vi "State Process.vi"(8 "error in (no error)":errorcluster, 11 "View Model":T1) -> (0 "error out":errorcluster, 3 "View Model":T1)   [LabVIEW 2017]
doc: "Provide processing current ATM controller state"
uses:
  View Model/Controls/View Model.ctl
  View Model/Controls/Shared Model.ctl
  Error Handler/Controls/Error Model.ctl
  Error Handler/Controls/Error Data.ctl
  Error Handler/Controls/Error Type.ctl
  Error Handler/Controls/Error Source.ctl
  Configuration/Controls/Config Model.ctl
  Configuration/Controls/Config CMD.ctl
  Configuration/Controls/Config Command.ctl
  Controls/Controller Model.ctl
  Controls/Controller Overhead.ctl
  Controls/Controller Transaction.ctl
  Controls/Controller State.ctl
  Configuration/Controls/Config Data Record.ctl
  Controls/Controller Message Selector.ctl
  Controls/Controller Message Type.ctl
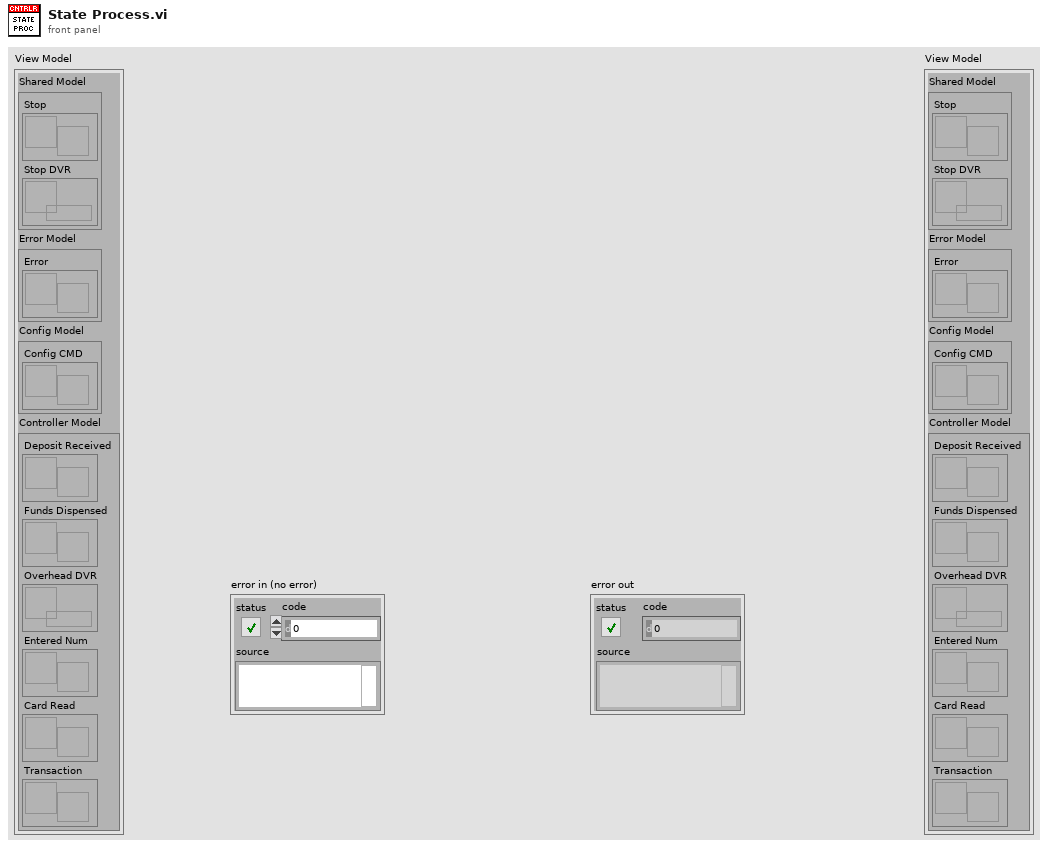
[diagram p1: front panel]
types:
  T1 = typedef "View Model.ctl" = cluster{"Shared Model":T2, "Error Model":T3, "Config Model":T4, "Controller Model":T5}
  T2 = typedef "Shared Model.ctl" = cluster{"Stop":refnum<user-event>, "Stop DVR":refnum<data-value>}
  T3 = typedef "Error Model.ctl" = cluster{"Error":refnum<user-event>}
  T4 = typedef "Config Model.ctl" = cluster{"Config CMD":refnum<user-event>}
  T5 = typedef "Controller Model.ctl" = cluster{"Deposit Received":refnum<user-event>, "Funds Dispensed":refnum<user-event>, "Overhead DVR":refnum<data-value>, "Entered Num":refnum<user-event>, "Card Read":refnum<user-event>, "Transaction":refnum<user-event>}
  T6 = typedef "Controller State.ctl" = enum16{"Idle", "Initial", "Login", "Balance Inquiry", "Deposit", "Withdrawal", "Fast Cash", "Terminate"}
  T7 = typedef "Controller Message Selector.ctl" = cluster{"Message Type":T8, "Dynamic Data":variant}
  T8 = typedef "Controller Message Type.ctl" = enum16{"Welcome", "Login", "Idle", "Invalid Login", "Terminate Session", "Deposit", "Withdrawal", "Fast Cash", "Withdrawal Complete", "Withdrawal Failed", "Balance"}
  T9 = typedef "Config Command.ctl" = enum16{"Read", "Search", "Update"}
  T10 = typedef "Config Data Record.ctl" = cluster{"Account Number":u32, "First Name":string, "Last Name":string, "Balance":dbl}
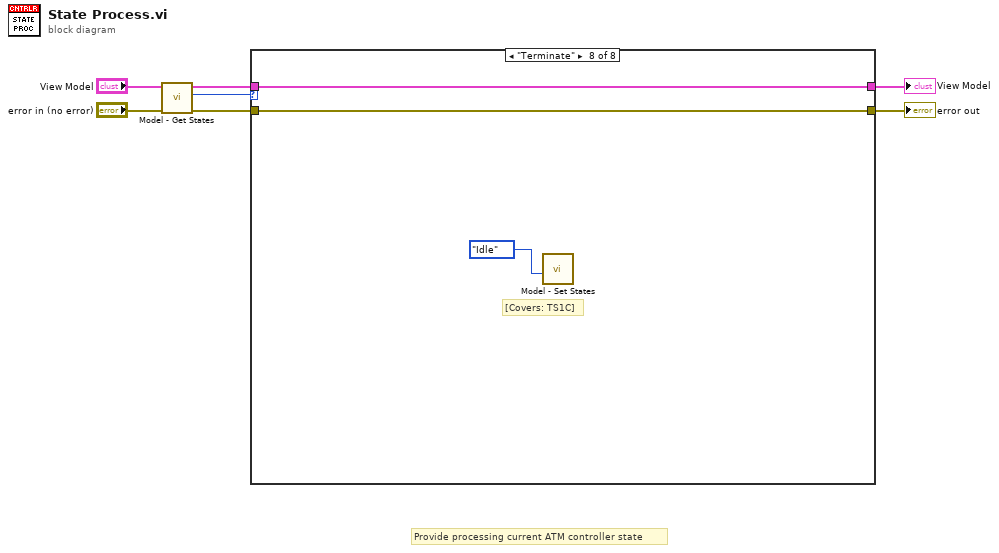
[diagram p0: block diagram]
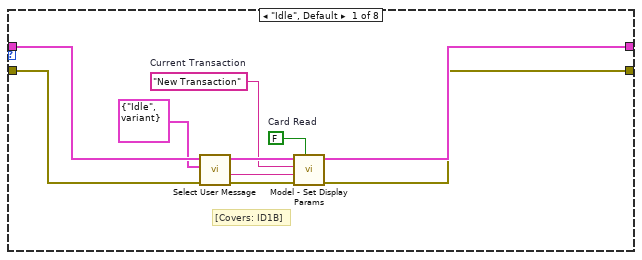
[diagram p2: hidden frame]
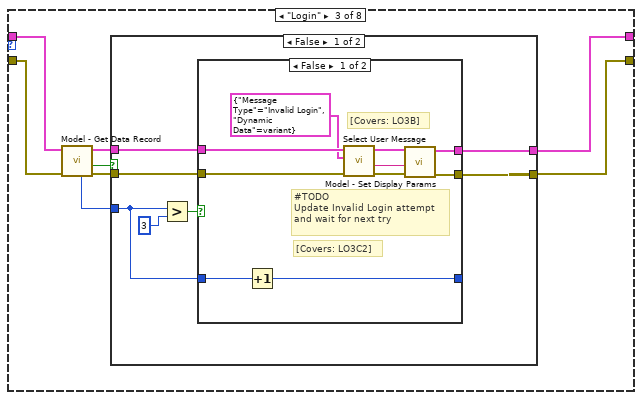
[diagram p4: hidden frame]
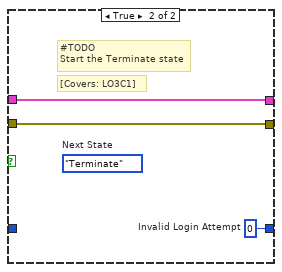
[diagram p5: hidden frame]
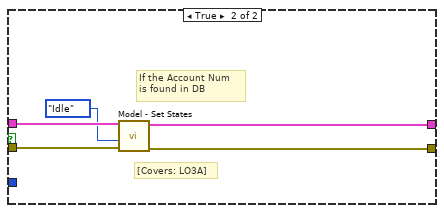
[diagram p6: hidden frame]
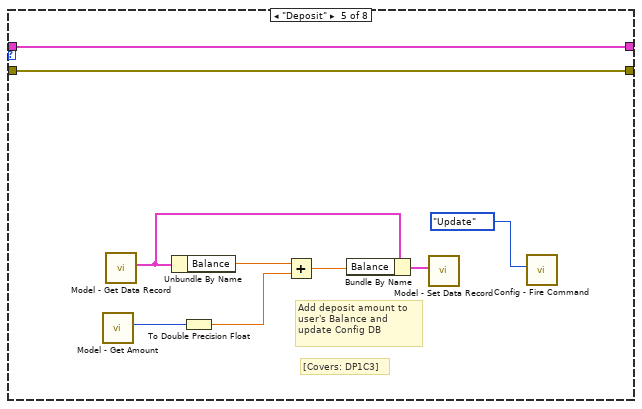
[diagram p8: hidden frame]
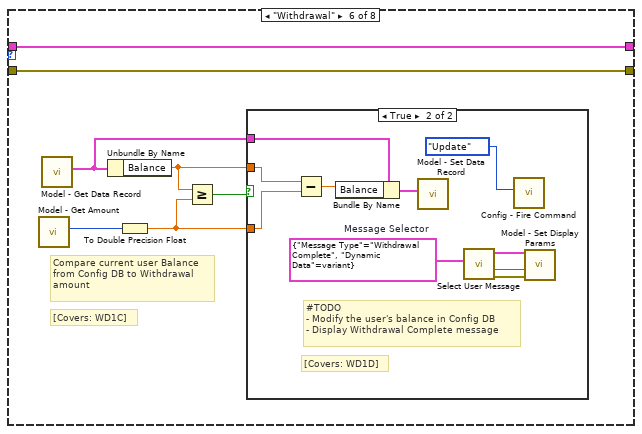
[diagram p9: hidden frame]
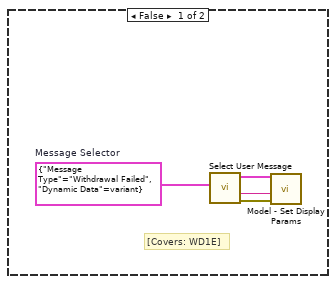
[diagram p10: hidden frame]
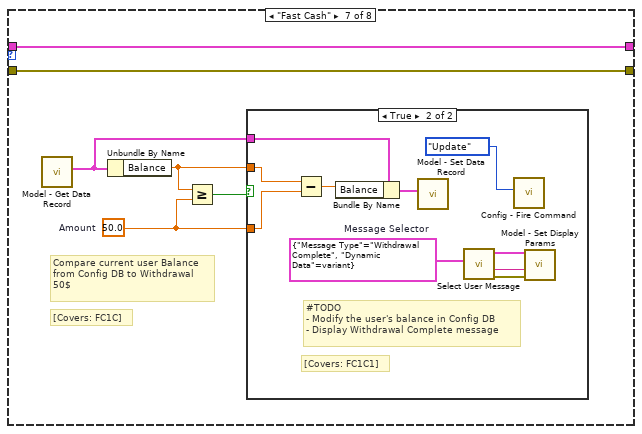
[diagram p11: hidden frame]
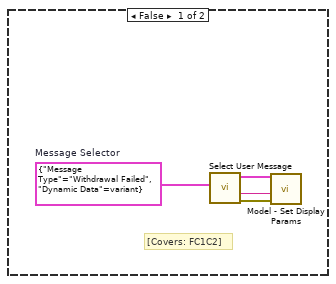
[diagram p12: hidden frame]
diagram:
  # "Provide processing current ATM controller state"
  n1 = call "Model - Get States.vi"("error in (no error)"="error in (no error)", "View Model"="View Model") -> ("error out"=w3:errorcluster, "Current State"=w5:T6, "View Model"=w4:T1)  [unwired: 6 in, 1 out]
  n2 = case shown="\"Terminate\"" w5 {
    tunnel: w4 -> [w16 w19 w26 w54 w63 w70 w90 w107]
    tunnel: w3 -> [w17 w18 w27 w53 w62 w69 w89 w106]
    tunnel: [w12 w19 w21 w54 w63 w70 w90 w107] -> w2
    tunnel: [w11 w18 w22 w53 w62 w69 w89 w106] -> w1
    frame "Idle", Default {
      w8 = FALSE  # Card Read
      w9 = "New Transaction"  # Current Transaction
      # "[Covers: ID1B]"
      n3 = call "Select User Message.vi"("error in (no error)"=w17, "Message Selector"=T7 {"Message Type"=enum."Idle", "Dynamic Data"=variant}, "View Model"=w16) -> ("error out"=w14:errorcluster, "Message"=w10:string, "View Model"=w13:T1)  [unwired: 6 in]
      n4 = call "Model - Set Display Params.vi"("Card Read"=w8, "error in (no error)"=w14, "Message"=w10, "Current Transaction"=w9, "View Model"=w13) -> ("error out"=w11:errorcluster, "View Model"=w12:T1)  [unwired: 5 in]
    }
    frame "Initial" {
    }
    frame "Login" {
      n5 = call "Model - Get Data Record.vi"("error in (no error)"=w27, "View Model"=w26) -> ("error out"=w23:errorcluster, "Account Found?"=w25:bool, "View Model"=w24:T1, "Invalid Login"=w20:u8)  [unwired: 5 in, 1 out]
      n6 = case shown="False" w25 {
        tunnel: w24 -> [w33 w51]
        tunnel: w23 -> [w34 w52]
        tunnel: [w32 w50] -> w22
        tunnel: [w31 w49] -> w21
        tunnel: w20 -> [w28 _]
        frame False {
          n7 = Greater?(x=w28, y=u8 3) -> (0:w30:bool)
          n8 = case shown="False" w30 {
            tunnel: w34 -> [w44 w47]
            tunnel: w33 -> [w43 w46]
            tunnel: [w40 w47] -> w32
            tunnel: [w39 w46] -> w31
            tunnel: w28 -> [w36 _]
            tunnel: [w35 w45] -> _
            frame False {
              # "[Covers: LO3C2]"
              # "#TODO\nUpdate Invalid Login attempt\nand wait for next try"
              # "[Covers: LO3B]"
              n9 = Increment(x=w36) -> (x+1=w35:u8)
              n10 = call "Select User Message.vi"("error in (no error)"=w44, "Message Selector"=T7 {"Message Type"=enum."Invalid Login", "Dynamic Data"=variant}, "View Model"=w43) -> ("error out"=w41:errorcluster, "Message"=w37:string, "View Model"=w42:T1)  [unwired: 6 in]
              n11 = call "Model - Set Display Params.vi"("error in (no error)"=w41, "Message"=w37, "View Model"=w42) -> ("error out"=w40:errorcluster, "View Model"=w39:T1)  [unwired: 7 in]
            }
            frame True {
              w45 = u8 0  # Invalid Login Attempt
              (unwired) Controller_State."Terminate"  # Next State
              # "[Covers: LO3C1]"
              # "#TODO\nStart the Terminate state"
            }
          }
        }
        frame True {
          # "[Covers: LO3A]"
          # "If the Account Num\nis found in DB"
          n12 = call "Model - Set States.vi"("error in (no error)"=w52, "Next State"=Controller_State."Idle", "View Model"=w51) -> ("error out"=w50:errorcluster, "View Model"=w49:T1)  [unwired: 7 in]
        }
      }
    }
    frame "Balance Inquiry" {
    }
    frame "Deposit" {
      # "[Covers: DP1C3]"
      # "Add deposit amount to\nuser's Balance and \nupdate Config DB"
      n13 = call "Model - Get Amount.vi"() -> ("Amount"=w60:u32)  [unwired: 9 in, 2 out]
      n14 = call "Model - Get Data Record.vi"() -> ("Data Record"=w58:T10)  [unwired: 7 in, 4 out]
      n15 = Unbundle By Name(w58) -> ("Balance"=w61:dbl)
      n16 = To Double Precision Float(number=w60) -> (double precision float=w59:dbl)
      n17 = Add(x=w61, y=w59) -> (x+y=w57:dbl)
      n18 = Bundle By Name(cluster=w58, "Balance"=w57) -> (w56:T10)
      n19 = call "Model - Set Data Record.vi"("Data Record"=w56) -> ()  [unwired: 9 in, 2 out]
      n20 = call "Config - Fire Command.vi"("CMD"=Config_Command."Update") -> ()  [unwired: 9 in, 2 out]
    }
    frame "Withdrawal" {
      # "[Covers: WD1C]"
      # "Compare current user Balance\nfrom Config DB to Withdrawal\namount"
      n21 = call "Model - Get Amount.vi"() -> ("Amount"=w68:u32)  [unwired: 9 in, 2 out]
      n22 = call "Model - Get Data Record.vi"() -> ("Data Record"=w64:T10)  [unwired: 7 in, 4 out]
      n23 = Unbundle By Name(w64) -> ("Balance"=w66:dbl)
      n24 = To Double Precision Float(number=w68) -> (double precision float=w65:dbl)
      n25 = Greater Or Equal?(x=w66, y=w65) -> (x >= y?=w67:bool)
      n26 = case shown="True" w67 {
        tunnel: w66 -> [_ w81]
        tunnel: w65 -> [_ w82]
        tunnel: w64 -> [_ w79]
        frame False {
          w71 = T7 {"Message Type"=enum."Withdrawal Failed", "Dynamic Data"=variant}  # Message Selector
          # "[Covers: WD1E]"
          n27 = call "Select User Message.vi"("Message Selector"=w71) -> ("error out"=w73:errorcluster, "Message"=w74:string, "View Model"=w72:T1)  [unwired: 8 in]
          n28 = call "Model - Set Display Params.vi"("error in (no error)"=w73, "Message"=w74, "View Model"=w72) -> ()  [unwired: 7 in, 2 out]
        }
        frame True {
          w75 = T7 {"Message Type"=enum."Withdrawal Complete", "Dynamic Data"=variant}  # Message Selector
          # "#TODO\n- Modify the user's balance in Config DB\n- Display Withdrawal Complete message"
          # "[Covers: WD1D]"
          n29 = Subtract(x=w81, y=w82) -> (x-y=w80:dbl)
          n30 = Bundle By Name(cluster=w79, "Balance"=w80) -> (w84:T10)
          n31 = call "Model - Set Data Record.vi"("Data Record"=w84) -> ()  [unwired: 9 in, 2 out]
          n32 = call "Select User Message.vi"("Message Selector"=w75) -> ("error out"=w77:errorcluster, "Message"=w78:string, "View Model"=w76:T1)  [unwired: 8 in]
          n33 = call "Config - Fire Command.vi"("CMD"=Config_Command."Update") -> ()  [unwired: 9 in, 2 out]
          n34 = call "Model - Set Display Params.vi"("error in (no error)"=w77, "Message"=w78, "View Model"=w76) -> ()  [unwired: 7 in, 2 out]
        }
      }
    }
    frame "Fast Cash" {
      w85 = 50.0  # Amount
      # "[Covers: FC1C]"
      # "Compare current user Balance\nfrom Config DB to Withdrawal\n50$"
      n35 = call "Model - Get Data Record.vi"() -> ("Data Record"=w86:T10)  [unwired: 7 in, 4 out]
      n36 = Unbundle By Name(w86) -> ("Balance"=w87:dbl)
      n37 = Greater Or Equal?(x=w87, y=w85) -> (x >= y?=w88:bool)
      n38 = case shown="True" w88 {
        tunnel: w87 -> [_ w101]
        tunnel: w85 -> [_ w102]
        tunnel: w86 -> [_ w99]
        frame False {
          w91 = T7 {"Message Type"=enum."Withdrawal Failed", "Dynamic Data"=variant}  # Message Selector
          # "[Covers: FC1C2]"
          n39 = call "Select User Message.vi"("Message Selector"=w91) -> ("error out"=w93:errorcluster, "Message"=w94:string, "View Model"=w92:T1)  [unwired: 8 in]
          n40 = call "Model - Set Display Params.vi"("error in (no error)"=w93, "Message"=w94, "View Model"=w92) -> ()  [unwired: 7 in, 2 out]
        }
        frame True {
          w95 = T7 {"Message Type"=enum."Withdrawal Complete", "Dynamic Data"=variant}  # Message Selector
          # "#TODO\n- Modify the user's balance in Config DB\n- Display Withdrawal Complete message"
          # "[Covers: FC1C1]"
          n41 = Subtract(x=w101, y=w102) -> (x-y=w100:dbl)
          n42 = Bundle By Name(cluster=w99, "Balance"=w100) -> (w104:T10)
          n43 = call "Model - Set Data Record.vi"("Data Record"=w104) -> ()  [unwired: 9 in, 2 out]
          n44 = call "Select User Message.vi"("Message Selector"=w95) -> ("error out"=w97:errorcluster, "Message"=w98:string, "View Model"=w96:T1)  [unwired: 8 in]
          n45 = call "Config - Fire Command.vi"("CMD"=Config_Command."Update") -> ()  [unwired: 9 in, 2 out]
          n46 = call "Model - Set Display Params.vi"("error in (no error)"=w97, "Message"=w98, "View Model"=w96) -> ()  [unwired: 7 in, 2 out]
        }
      }
    }
    frame "Terminate" {
      # "[Covers: TS1C]"
      n47 = call "Model - Set States.vi"("Next State"=Controller_State."Idle") -> ()  [unwired: 9 in, 2 out]
    }
  }
  "View Model" <- w2
  "error out" <- w1
